vi "DHE_get_controller_info.vi"(0 "fd":i32, 11 "error in (no error)":errorcluster) -> (4 "fd":i32, 6 "info":string, 8 "error_code":i32, 15 "error out":errorcluster)   [LabVIEW 2016]
doc: "This VI closes the I/O interface with the instrument."
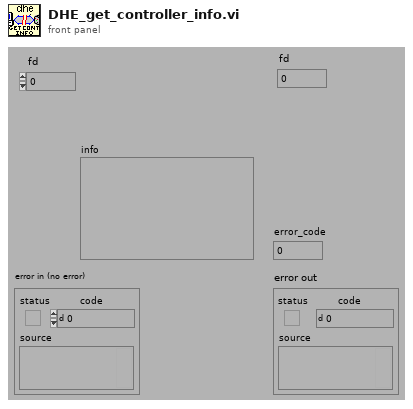
[diagram p1: front panel]
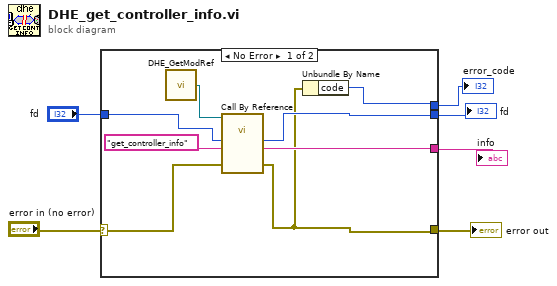
[diagram p0: block diagram]
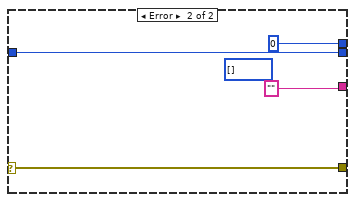
[diagram p2: hidden frame]
diagram:
  n1 = case shown="No Error" "error in (no error)" {
    selector: "error in (no error)" -> [w11 w16]
    tunnel: "fd" -> [w12 w18]
    tunnel: [w8 0] -> w5
    tunnel: [w7 w16] -> w4
    tunnel: [w10 w18] -> w3
    tunnel: [w9 "" ("str result")] -> w1
    frame No Error {
      n2 = call "DHE_GetModRef.vi"() -> ("DHE_ModRef"=w14:refnum<vi>)  [unwired: 9 out]
      n3 = call-by-ref "?"(reference=w14, "error in (no error)"=w11, "function"="get_controller_info", "fd in"=w12) -> ("error out"=w7:errorcluster, "str result"=w9:string, "fd out"=w10:i32)  [unwired: 6 in, 3 out]
      n4 = Unbundle By Name(w7) -> ("code"=w8:i32)
    }
    frame Error {
      (unwired) u16[] [] ("info")
    }
  }
  "error out" <- w4
  "error_code" <- w5
  "fd" <- w3
  "info" <- w1
